vi "VelocityPID.vi"() -> ()   [LabVIEW 2016]
uses:
  <vilib>/MakerHub/LINX/Public/Utilities/Open Serial.vi
  <vilib>/addons/control/pid/pid.llb/PID (DBL).vi
  <vilib>/MakerHub/LINX/LMH-LINX.lvlib
  <vilib>/addons/control/pid/NI_PID_pid.lvlib
panel:
  in  "T":u32
  out "Loop Rate (Hz)":u32
  in  "setpoint":dbl format="%.2f"
  out "Set-Point - RPM":dynamicdata(graph)
  out "Voltage":dbl(graph)
  in  "IN 4":u8
  in  "IN3":u8
  in  "PWM Channel":u8
  in  "stop":bool
  in  "Source Voltage":dbl
  in  "Number of pulses":i32
  in  "output range":cluster{"output high":dbl, "output low":dbl}={"output high"=100.0, "output low"=-100.0} {"output low" format="%.2f"; "output high" format="%.2f"}
  in  "PID gains":T1={"proportional gain (Kc)"=1.0, "integral time (Ti, min)"=0.01, "derivative time (Td, min)"=0.0} {"derivative time (Td, min)" format="%.3f"; "integral time (Ti, min)" format="%.3f"; "proportional gain (Kc)" format="%.3f"}
  in  "Serial Port":refnum<visa-resource-name>="N/A"
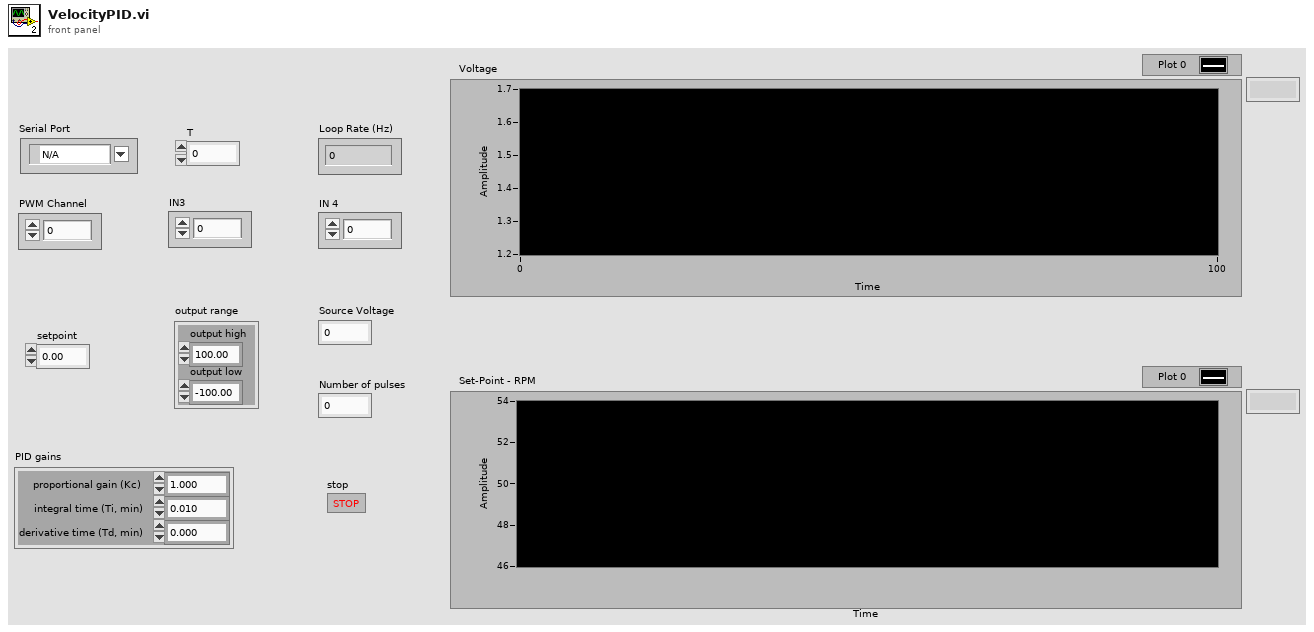
[diagram p1: front panel]
types:
  T1 = cluster{"proportional gain (Kc)":dbl, "integral time (Ti, min)":dbl, "derivative time (Td, min)":dbl}
  T2 = typedef "LMH-LINX.lvlib/LINX Ref.ctl" = cluster{"IO":T3, "Interface":T4, "LINX Device Config":T5}
  T3 = typedef "LMH-LINX.lvlib/Platform.ctl" = enum16{"Remote", "Local"}
  T4 = typedef "LMH-LINX.lvlib/Interface.ctl" = enum16{"Serial", "TCP"}
  T5 = typedef "LMH-LINX.lvlib/Device.lvlib/LINX Device Config.ctl" = cluster{"Interface":T4, "COM Port":refnum<visa-resource-name>, "TCP Configuration":T6, "Device Family":u8, "Device ID":u8, "Device Name":string, "TCP Ref":refnum<k5>, "Channels":T7}
  T6 = typedef "LMH-LINX.lvlib/Device.lvlib/TCP Config.ctl" = cluster{"IP Address":string, "Port":u16}
  T7 = typedef "LMH-LINX.lvlib/Channels.ctl" = cluster{"DI":u8[], "DO":u8[], "AI":u8[], "AO":u8[], "PWM":u8[], "QE":u8[], "UART":u8[], "I2C 2":u8[], "SPI":u8[], "CAN":u8[], "Servo":u8[], "AI Ref (V)":dbl, "AI Resolution (Bits)":u8, "AO Ref (V)":dbl, "AO Resolution (Bits)":u8}
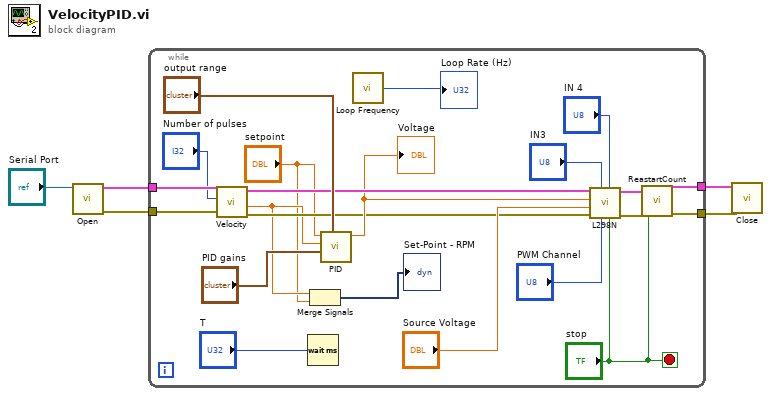
[diagram p0: block diagram]
diagram:
  n1 = call-poly <vilib>:"Open.vi"("Serial Port"="Serial Port") -> ("Error Out"=w4:errorcluster, "LINX Resource"=w5:T2)  [unwired: 8 in, 1 out]
  n2 = while {
    tunnel: w5 -> [w27]
    tunnel: w4 -> [w26]
    tunnel: [w16] -> w2
    tunnel: [w15] -> w1
    stop <- "stop" stop-if-true
    n3 = call "Velocity.vi"("Error In"=w26, "Number of pulses"="Number of pulses", "LINX Resource IN"=w27) -> ("Error Out"=w10:errorcluster, "RPM"=w9:dbl, "LINX Resource OUT"=w22:T2)  [unwired: 3 in, 3 out]
    n4 = Wait (ms)(milliseconds to wait="T") -> ()  [unwired: 1 out]
    n5 = Merge Signals(w9, "setpoint") -> (→"Set-Point - RPM":dynamicdata)
    n6 = call-poly <vilib>:"PID.vi"("output range"="output range", "PID gains"="PID gains", "process variable"=w9, "setpoint"="setpoint") -> ("output"=w14:dbl)  [unwired: 6 in, 1 out]
    "Voltage" <- w14
    n7 = call <vilib>:"Loop Frequency.vi"() -> ("Loop Rate (Hz)"=→"Loop Rate (Hz)":u32)
    n8 = call "L298N.vi"("Turn Off"="stop", "IN 4"="IN 4", "PWM Channel"="PWM Channel", "IN3"="IN3", "Error In"=w10, "Source Voltage"="Source Voltage", "Voltage"=w14, "LINX Resource IN"=w22) -> ("Error Out"=w17:errorcluster, "LINX Resource OUT"=w18:T2)  [unwired: 2 in]
    n9 = call "ReastartCount.vi"("Error In"=w17, "Activate"="stop", "LINX Resource IN"=w18) -> ("Error Out"=w15:errorcluster, "LINX Resource OUT"=w16:T2)  [unwired: 7 in]
  }
  n10 = call <vilib>:"Close.vi"("Error In"=w1, "LINX Resource"=w2) -> ()  [unwired: 9 in, 1 out]
